vi "SwipeMenu Demo.vi"() -> ()   [LabVIEW 2020]
uses:
  Swipe Menu Class/SwipeMenu.lvclass
panel:
  out "Button Pressed":string
  # "Swipe Menu"
  # "Note: You will need the QControl Toolkit to run this."
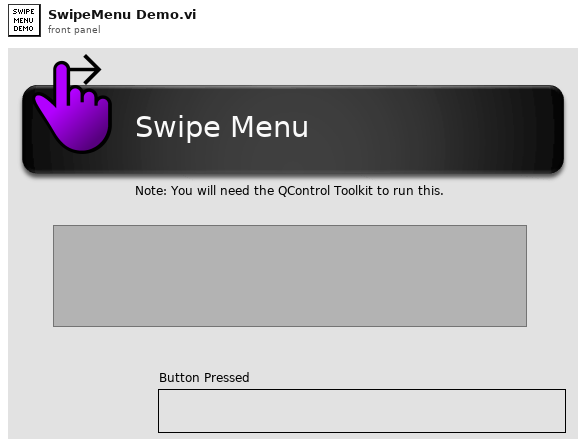
[diagram p1: front panel]
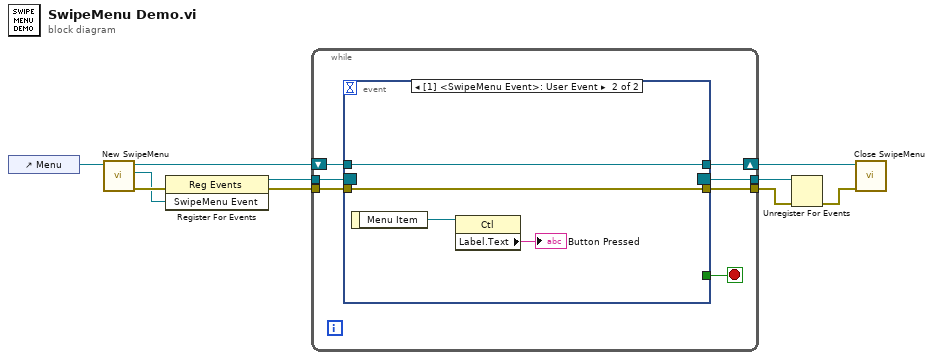
[diagram p0: block diagram]
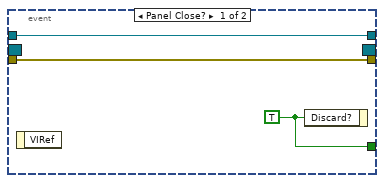
[diagram p2: hidden frame]
diagram:
  n1 = control-ref of="Menu"() -> (w8:refnum<vi>)
  n2 = call "New SwipeMenu.vi"("Reference"=w8) -> ("error out"=w7:errorcluster, "SwipeMenu Event"=w5:refnum<user-event>, "SwipeMenu out"=w9:refnum<class "SwipeMenu.lvclass">)  [unwired: 8 in]
  n3 = register-events(error in=w7, w5) -> (reference out=w4:refnum<event-registration>, error out=w6:errorcluster)  [unwired: 1 in]
  n4 = while {
    shift-right: [w16] -> w10
    shift-left: w9 -> [w15]
    tunnel: w6 -> [w13]
    tunnel: [w14] -> w2
    tunnel: w4 -> [w12]
    tunnel: [w11] -> w3
    stop <- w17 stop-if-true
    n5 = event shown="[1] <SwipeMenu Event>: User Event" {
      selector: w12 -> [_ _]
      dyn-events: [_ _] -> w11
      timeout: _ -> [_ _]
      tunnel: [w20 _] -> w17
      tunnel: [w19 w24] -> w16
      tunnel: w15 -> [w19 w24]
      tunnel: [w18 w23] -> w14
      tunnel: w13 -> [w18 w23]
      event Panel Close? {
        w20 = TRUE ("Discard?")
        n6 = event-data() -> ()  [unwired: 1 in, 1 out]
        n7 = event-data("Discard?"=w20) -> ()  [unwired: 1 in, 1 out]
      }
      event User Event {
        n8 = event-data() -> ("Menu Item"=w22:refnum<vi>)  [unwired: 1 in]
        n9 = property class="Ctl"(reference=w22) -> ("Label.Text"=→"Button Pressed":string)  [unwired: 1 in, 2 out]
      }
    }
  }
  n10 = Unregister For Events(event registration refnum=w3, error in=w2) -> (error out=w1:errorcluster)
  n11 = call "Close SwipeMenu.vi"("error in (no error)"=w1, "SwipeMenu in"=w10) -> ()  [unwired: 9 in, 1 out]
